vi "Pod Code.vi"   [LabVIEW 2017]
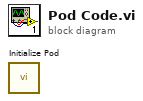
[diagram p0: block diagram]
diagram:
  n1 = call "Initialize Pod.vi"() -> ()  [unwired: 10 in, 2 out]
